vi "Gen - Add Time.vi"(8 "Error In":errorcluster, 10 "#days":i32=1, 11 "Time In":timestamp=timestamp(3635049600 s since 1904-01-01)) -> (0 "Error Out":errorcluster, 3 "Time Out":timestamp)   [LabVIEW 2020]
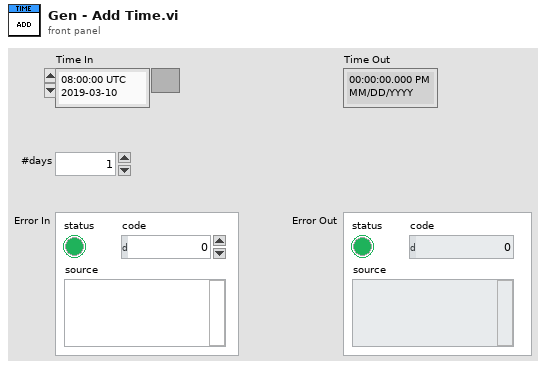
[diagram p1: front panel]
types:
  T1 = typedef "LVDateTimeRec.ctl" = cluster{"fractional second":dbl, "second":i32, "minute":i32, "hour":i32, "day of month":i32, "month":i32, "year":i32, "day of week":i32, "day of year":i32, "DST":i32}
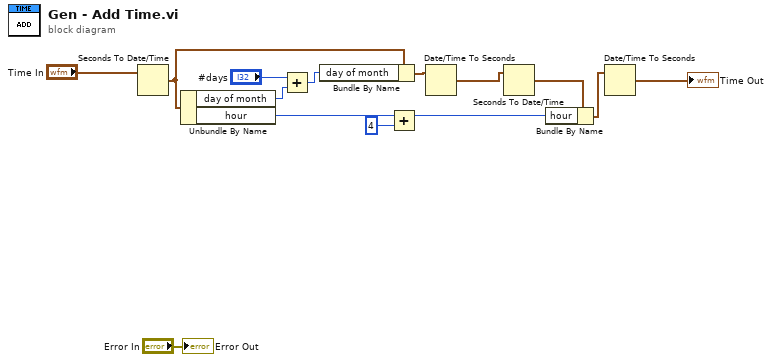
[diagram p0: block diagram]
diagram:
  n1 = Seconds To Date/Time(time stamp (now)="Time In") -> (date time rec=w12:T1)  [unwired: 1 in]
  n2 = Unbundle By Name(w12) -> ("day of month"=w11:i32, "hour"=w5:i32)
  n3 = Add(x="#days", y=w11) -> (x+y=w10:i32)
  n4 = Bundle By Name(cluster=w12, "day of month"=w10) -> (w9:T1)
  n5 = Add(x=w5, y=4) -> (x+y=w2:i32)
  n6 = Date/Time To Seconds(2:w9) -> (0:w7:timestamp)  [unwired: 1 in]
  n7 = Seconds To Date/Time(time stamp (now)=w7) -> (date time rec=w6:T1)  [unwired: 1 in]
  n8 = Bundle By Name(cluster=w6, "hour"=w2) -> (w4:T1)
  n9 = Date/Time To Seconds(2:w4) -> (0:→"Time Out":timestamp)  [unwired: 1 in]
  "Error Out" <- "Error In"
